vi "Logged_Data_real_Global.vi"() -> ()   [LabVIEW 2010]
panel:
  in  "Data":dbl[][](array[numeric]) format="%.2f"
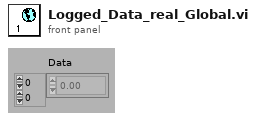
[diagram p1: front panel]
diagram:
